vi "Fibonacci series.vi"() -> ()   [LabVIEW 2020]
panel:
  out "iteration count":dbl
  out "fibonacci series":dbl
  in  "total count":dbl
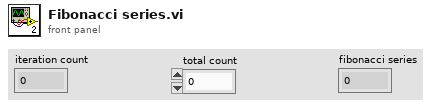
[diagram p1: front panel]
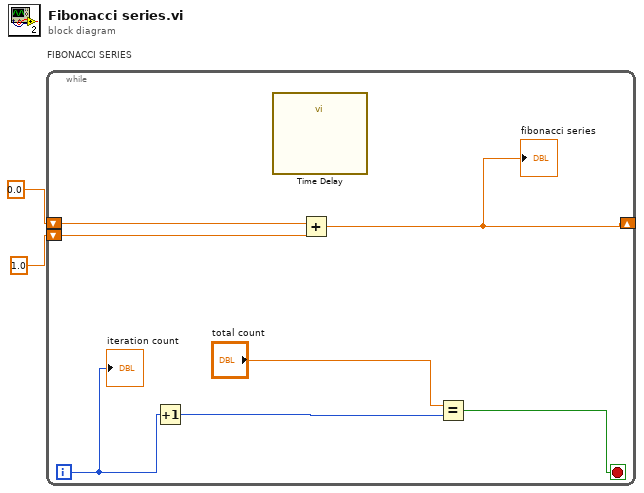
[diagram p0: block diagram]
diagram:
  n1 = while "FIBONACCI SERIES" {
    shift-right: [w4] -> _
    shift-left: 0.0 -> [w6]
    shift-left: 1.0 -> [w5]
    i -> [w3]
    stop <- w7 stop-if-true
    n2 = Increment(x=w3) -> (x+1=w9:i32)
    n3 = call "Time Delay"() -> ()  [unwired: 11 in, 1 out]
    n4 = Add(x=w6, y=w5) -> (x+y=w4:dbl)
    "fibonacci series" <- w4
    n5 = Equal?(x="total count", y=w9) -> (x = y?=w7:bool)
    "iteration count" <- w3
  }
